vi "Quiz #3.vi"() -> ()   [LabVIEW 2017]
uses:
  Controlaleluya.ctl
  Maquinaestaleluya.ctl
  Control 2maqinestaaleluya.ctl
panel:
  out "array w/ subset deleted 4":string[][](array[string])
  out "spreadsheet string 4":string
  out "before substring 12":string
  out "match substring 12":string
  out "after substring 12":string
  out "text 8":string
  out "array 8":string[][](array[string])
  out "C.V 8":u8[](array[numeric])
  out "stop 16":bool
  out "C.V 7":u8[](array[numeric])
  out "stop 15":bool
  out "text 7":string
  out "array 7":string[][](array[string])
  out "element 8":string
  out "before substring 11":string
  out "match substring 11":string
  out "after substring 11":string
  out "element 7":string
  out "before substring 10":string
  out "match substring 10":string
  out "after substring 10":string
  in  "stop 14":bool
  in  "stop 13":bool
  out "Tab Control 2":enum32{"Loguin", "Usuarios", "Admin"}(tab)
  in  "Loguin 2":bool
  in  "Contraseña 4":string
  in  "Usuario 4":string
  in  "Nombre 4":string
  in  "Clave 4":string
  in  "Aceptar 4":bool
  out "OK Button 3":bool
  in  "Ingresar 2":bool
  in  "Borrar 2":bool
  in  "Clave/ingress 4":string
  in  "Usua/Ingress 4":string
  in  "Usuarios D/B 4":string[](array[string])
  out "mayu 2":i32
  out "min 2":i32
  in  "Salir 2":bool
  out "appended path 2":path
  in  "stop 3":bool
  in  "Salir":bool
  out "array 2":string[][](array[string])
  out "text 2":string
  out "appended path":path
  out "array w/ subset deleted":string[][](array[string])
  out "spreadsheet string":string
  out "after substring 3":string
  out "match substring 3":string
  out "before substring 3":string
  out "C.V":u8[](array[numeric])
  out "stop 4":bool
  out "C.V 2":u8[](array[numeric])
  out "mayu":i32
  out "min":i32
  out "stop 2":bool
  out "after substring 2":string
  out "match substring 2":string
  out "before substring 2":string
  out "element 2":string
  out "after substring":string
  out "match substring":string
  out "before substring":string
  out "element":string
  out "array":string[][](array[string])
  out "text":string
  in  "stop":bool
  out "Tab Control":enum32{"Loguin", "Usuarios", "Admin"}(tab)
  in  "Usuario":string
  in  "Contraseña":string
  in  "Loguin":bool
  out "OK Button":bool
  in  "Clave":string
  in  "Nombre":string
  in  "Aceptar":bool
  out "OK Button 2":bool
  in  "Ingresar":bool
  in  "Usua/Ingress":string
  in  "Clave/ingress":string
  in  "Borrar":bool
  in  "Usuarios D/B":string[](array[string])
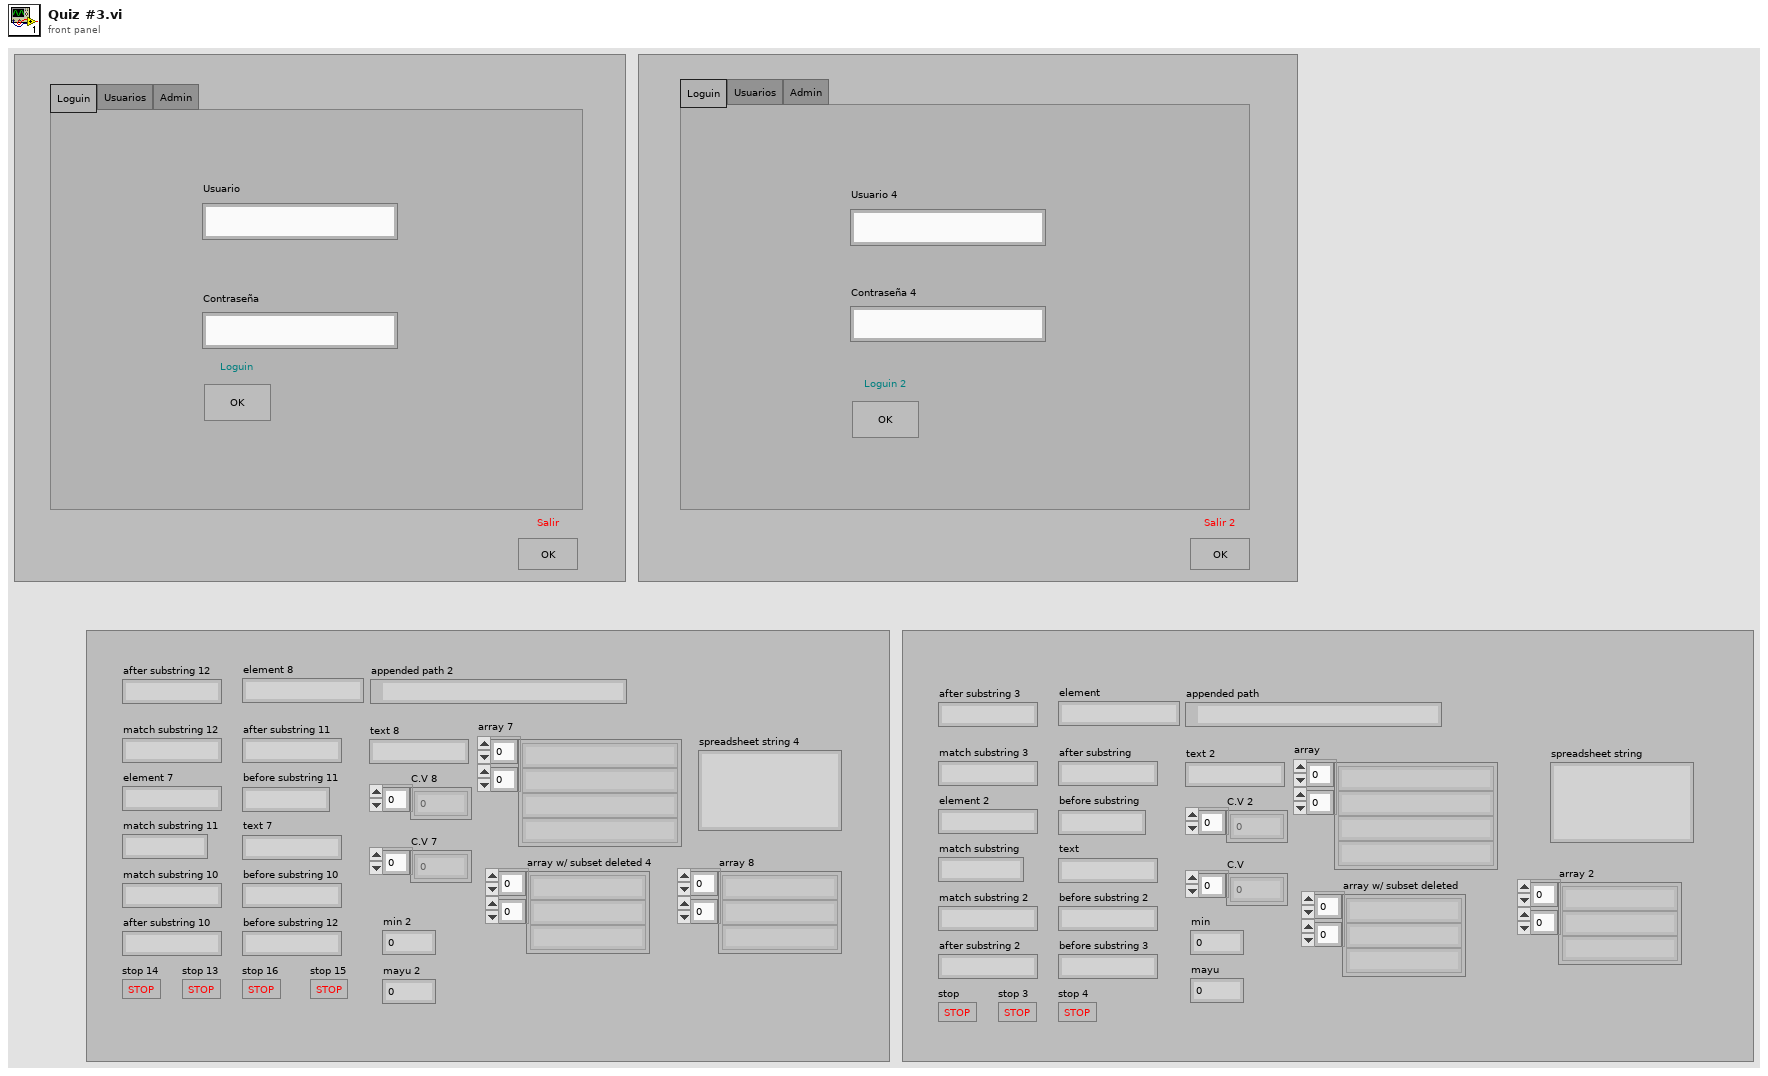
[diagram p1: front panel]
types:
  T1 = enum16{"open", "replace", "create", "open or create", "replace or create", "replace or create with confirmation"}
  T2 = typedef "Controlaleluya.ctl" = enum16{"Loguin", "Usuarios", "Admin"}
  T3 = typedef "Maquinaestaleluya.ctl" = enum16{"Control", "V.Usuario/Contraseña", "V.entre 8 y 16", "V.min y MAY", "ingresar"}
  T4 = typedef "Control 2maqinestaaleluya.ctl" = enum16{"Control", "V.Usuario/Contraseña", "V.Entre 8 y 16", "V.min y MAY", "Aceptar"}
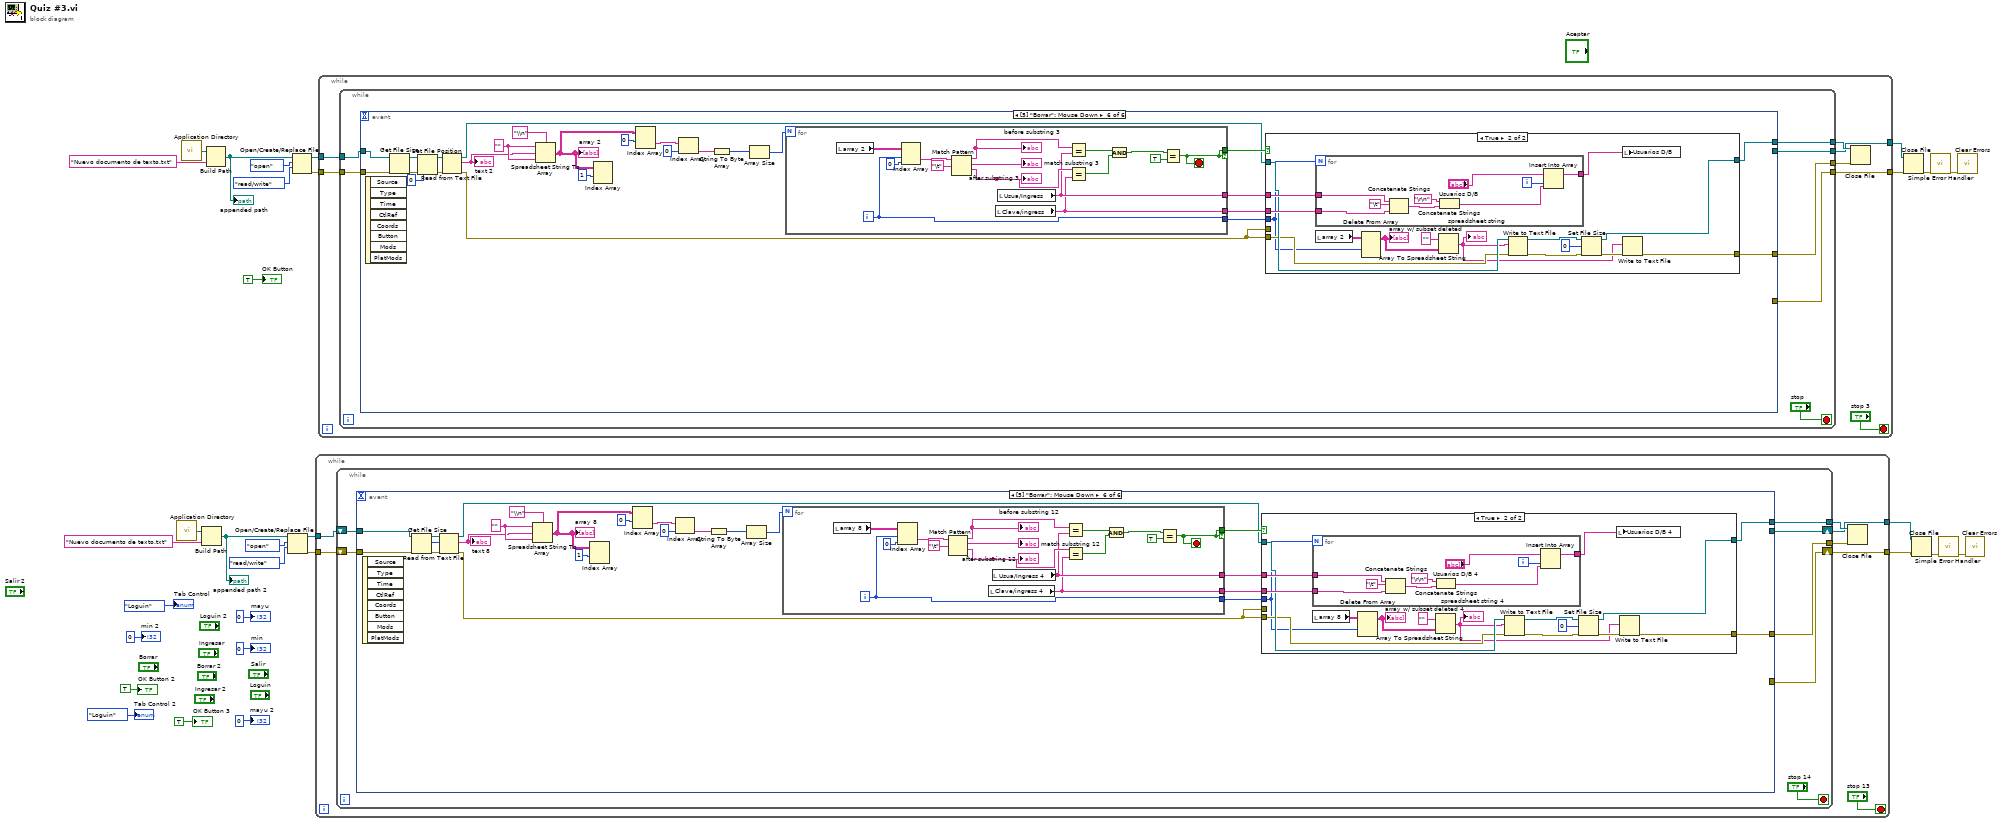
[diagram p0: block diagram]
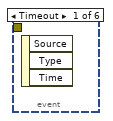
[diagram p2: hidden frame]
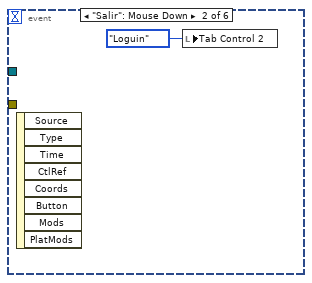
[diagram p3: hidden frame]
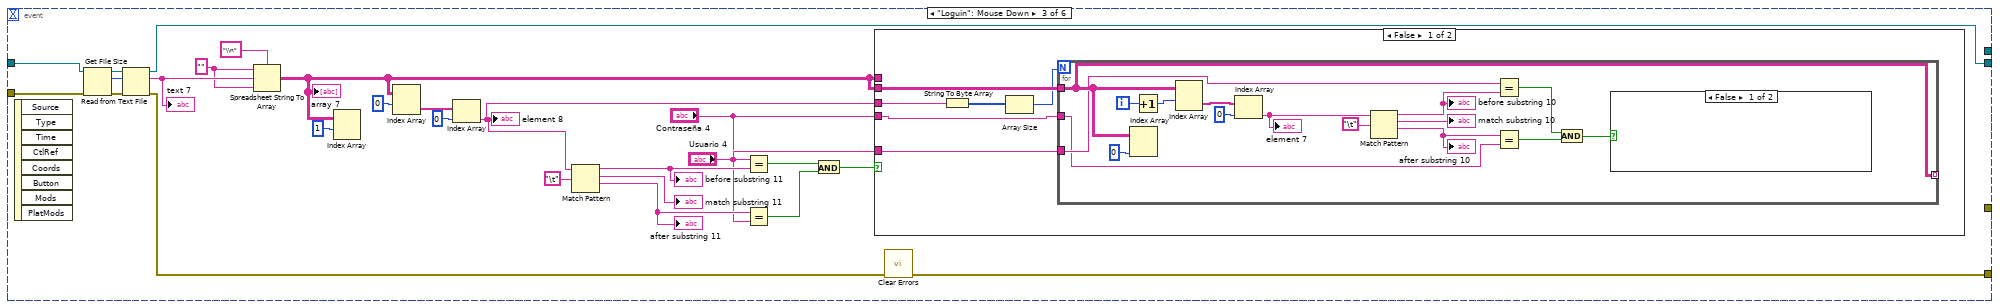
[diagram p4: hidden frame]
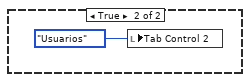
[diagram p5: hidden frame]
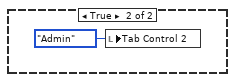
[diagram p6: hidden frame]
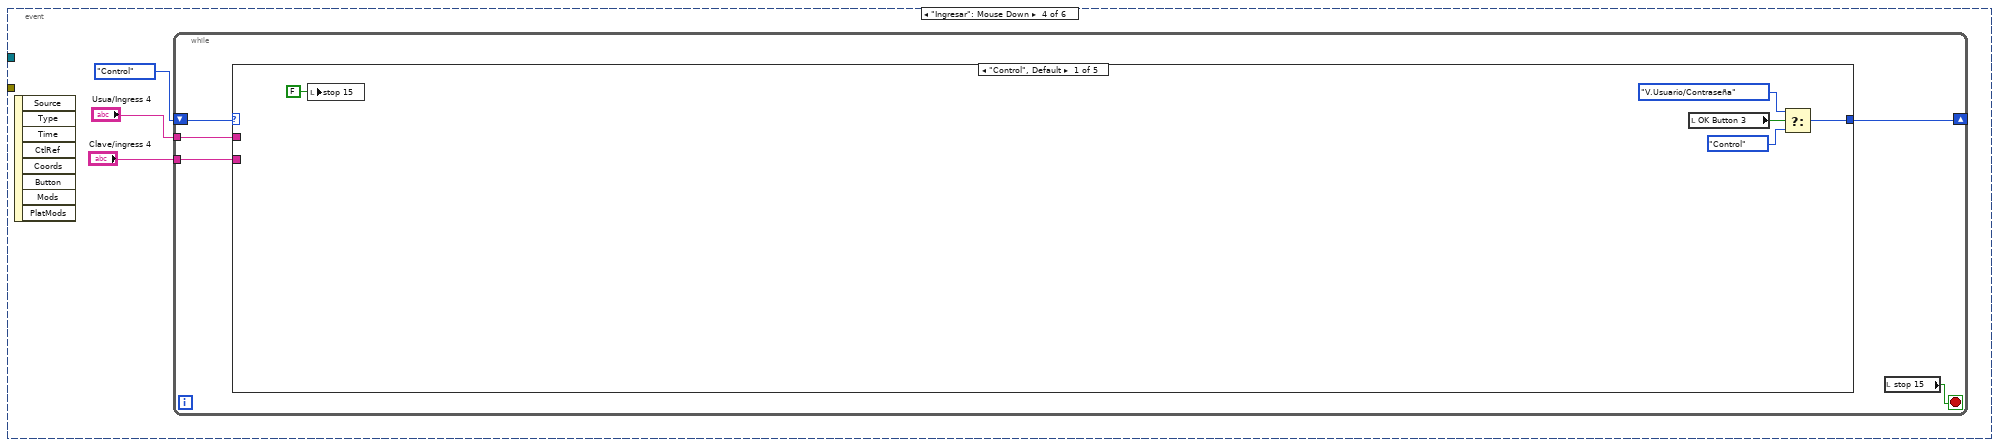
[diagram p7: hidden frame]
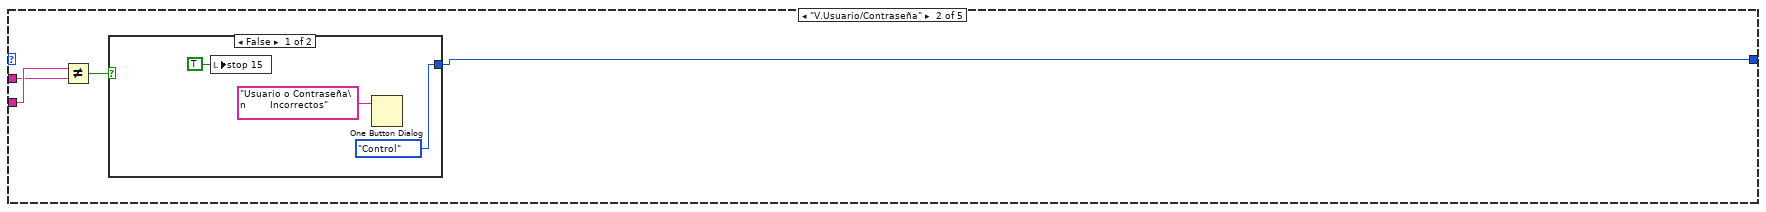
[diagram p8: hidden frame]
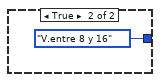
[diagram p9: hidden frame]
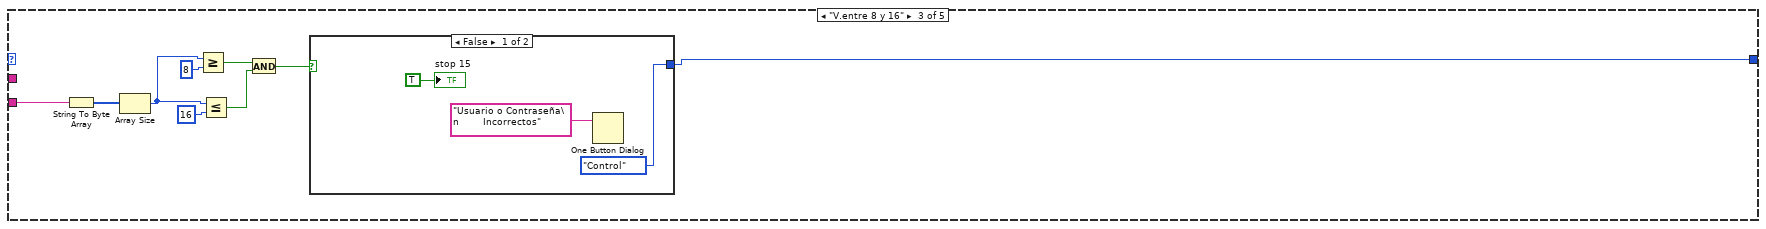
[diagram p10: hidden frame]
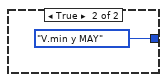
[diagram p11: hidden frame]
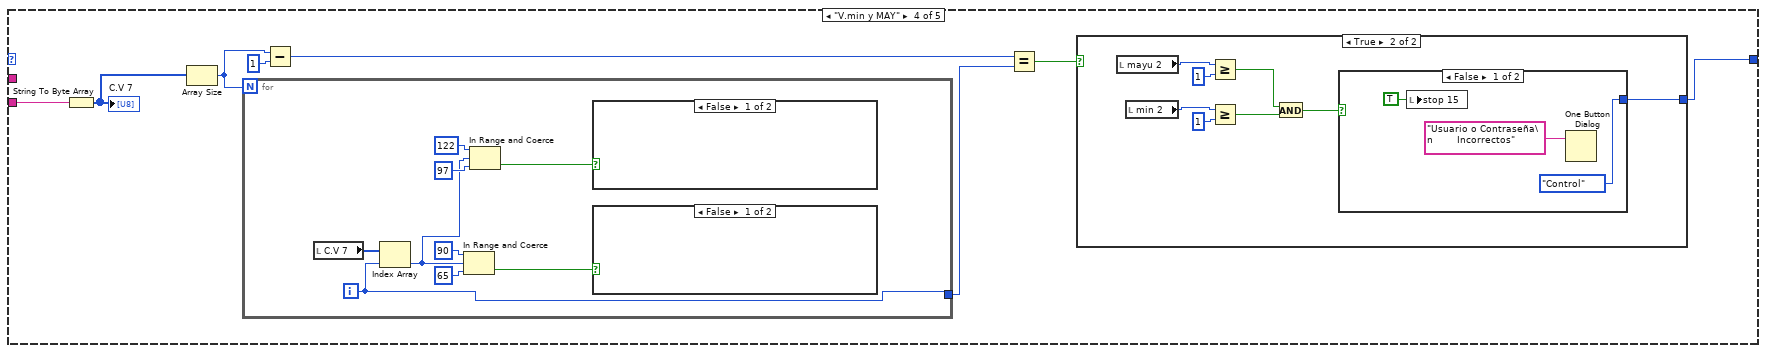
[diagram p12: hidden frame]
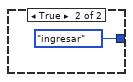
[diagram p14: hidden frame]
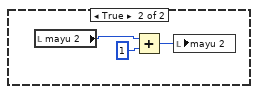
[diagram p15: hidden frame]
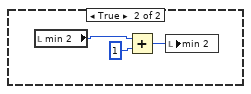
[diagram p16: hidden frame]
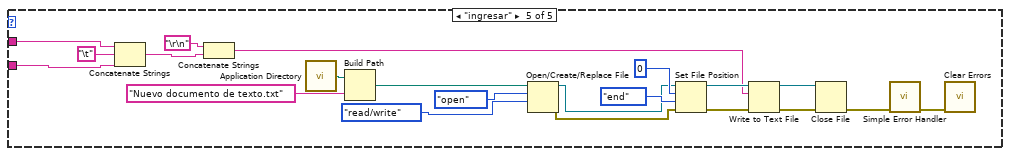
[diagram p17: hidden frame]
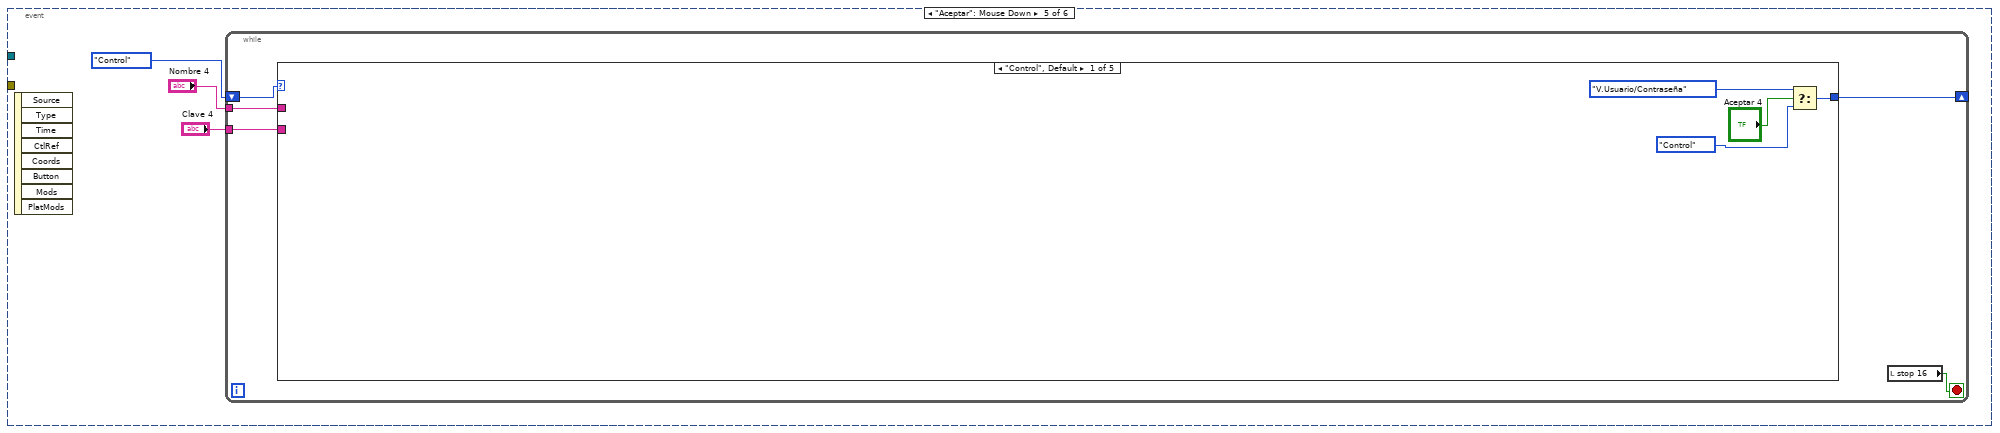
[diagram p18: hidden frame]
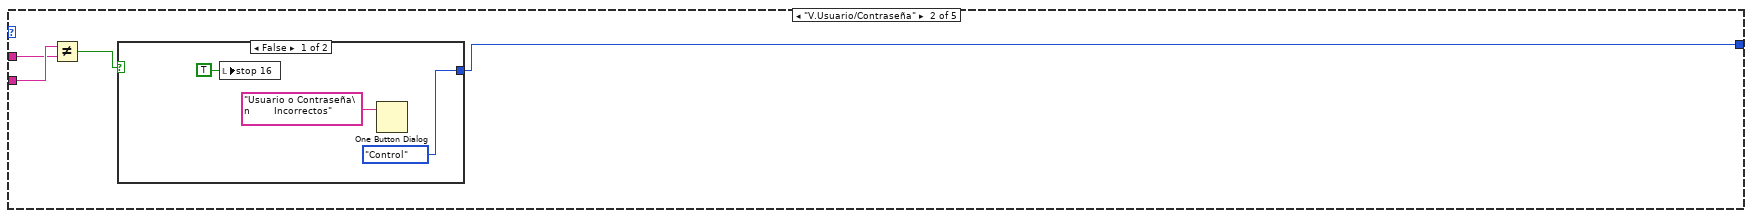
[diagram p19: hidden frame]
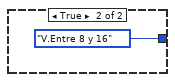
[diagram p20: hidden frame]
diagram:
  n1 = call <vilib>:"Application Directory.vi"() -> ("Application Directory"=w11:path)
  n2 = call <vilib>:"Application Directory.vi"() -> ("Application Directory"=w24:path)
  n3 = Build Path(base path=w11, name or relative path="Nuevo documento de texto.txt") -> (appended path=w13:path)
  "appended path 2" <- w13
  n4 = Build Path(base path=w24, name or relative path="Nuevo documento de texto.txt") -> (appended path=w22:path)
  "appended path" <- w22
  n5 = Open/Create/Replace File(file path (use dialog)=w13, operation (0:open)=T1."open", access (0:read/write)=enum16{"read/write", "read-only", "write-only"}."read/write") -> (refnum out=w5:refnum<file>, error out=w4:errorcluster)  [unwired: 3 in, 1 out]
  n6 = Open/Create/Replace File(file path (use dialog)=w22, operation (0:open)=T1."open", access (0:read/write)=enum16{"read/write", "read-only", "write-only"}."read/write") -> (refnum out=w26:refnum<file>, error out=w25:errorcluster)  [unwired: 3 in, 1 out]
  n7 = while {
    tunnel: w5 -> [w38]
    tunnel: w4 -> [w37]
    tunnel: [w34] -> w2
    tunnel: [w33] -> w3
    stop <- "stop 13" stop-if-true
    n8 = while {
      tunnel: [w44] -> w36
      tunnel: [w43] -> w35
      shift-right: [w40] -> w33
      shift-left: w38 -> [w42]
      shift-right: [w41] -> w34
      shift-left: w37 -> [w39]
      stop <- "stop 14" stop-if-true
      n9 = event shown="[5] \"Borrar\": Mouse Down" {
        selector: _ -> [_ _ _ _ _ _]
        dyn-events: _ -> [_ _ _ _ _ _]
        timeout: _ -> [_ _ _ _ _ _]
        tunnel: [_ _ w69 _ _ _] -> w41
        tunnel: [_ _ w57 _ _ _] -> w40
        tunnel: w42 -> [_ _ w51 _ _ w293]
        tunnel: w39 -> [_ _ w53 _ _ w292]
        tunnel: [_ _ _ _ _ w286] -> w44
        tunnel: [_ _ _ _ _ w285] -> w43
        event Timeout {
          n10 = event-data() -> ()  [unwired: 1 in, 3 out]
        }
        event "Salir": Mouse Down {
          n11 = event-data() -> ()  [unwired: 1 in, 8 out]
          n12 = local write "Tab Control 2"(Controlaleluya."Loguin") -> ()
        }
        event "Loguin": Mouse Down {
          w59 = "" ("array type (2D Dbl)")
          n13 = event-data() -> ()  [unwired: 1 in, 8 out]
          n14 = Get File Size(file=w51, error in=w53) -> (refnum out=w52:refnum<file>, size (in bytes)=w71:i64, 0:w72:errorcluster)
          n15 = Read from Text File(file (use dialog)=w52, count=w71, error in=w72) -> (refnum out=w57:refnum<file>, text=w68:string, error out=w70:errorcluster)  [unwired: 1 in, 1 out]
          "text 7" <- w68
          n16 = Spreadsheet String To Array(delimiter (Tab)="\\n", format string=w59, spreadsheet string=w68, array type (2D Dbl)=w59) -> (array=w50:string[][])
          "array 7" <- w50
          n17 = Index Array(array=w50, index (row)=1 ("index")) -> ()  [unwired: 1 in, 1 out]
          n18 = Index Array(array=w50, index (row)=0) -> (element=w64:string[])  [unwired: 1 in]
          n19 = Index Array(array=w64, index=0) -> (element=w56:string)
          "element 8" <- w56
          n20 = Match Pattern(string=w56, regular expression="\t") -> (before substring=w58:string, match substring=→"match substring 11":string, after substring=w60:string)  [unwired: 1 in, 1 out]
          "before substring 11" <- w58
          "after substring 11" <- w60
          n21 = Equal?(x="Usuario 4", y=w58) -> (x = y?=w49:bool)
          n22 = Equal?(x=w60, y="Contraseña 4") -> (x = y?=w48:bool)
          n23 = And(x=w49, y=w48) -> (x .and. y?=w47:bool)
          n24 = case shown="False" w47 {
            tunnel: w50 -> [_ _]
            tunnel: w50 -> [w78 _]
            tunnel: w56 -> [w77 _]
            tunnel: "Usuario 4" -> [w75 _]
            tunnel: "Contraseña 4" -> [w74 _]
            frame False {
              n25 = String To Byte Array(string=w77) -> (unsigned byte array=w76:u8[])
              n26 = Array Size(array=w76) -> (size(s)=w73:i32)
              n27 = for {
                N: w73 -> [_]
                tunnel: w78 -> [w83]
                tunnel: [w83] -> _ mode=indexing
                tunnel: w75 -> [w82]
                tunnel: w74 -> [w81]
                i -> [w80]
                n28 = Index Array(array=w83, index (col)=0) -> ()  [unwired: 1 in, 1 out]
                n29 = Increment(x=w80) -> (x+1=w79:i32)
                n30 = Index Array(array=w83, index (row)=w79) -> (element=w92:string[])  [unwired: 1 in]
                n31 = Index Array(array=w92, index=0) -> (element=w91:string)
                "element 7" <- w91
                n32 = Match Pattern(string=w91, regular expression="\t") -> (before substring=w89:string, match substring=→"match substring 10":string, after substring=w87:string)  [unwired: 1 in, 1 out]
                "before substring 10" <- w89
                "after substring 10" <- w87
                n33 = Equal?(x=w82, y=w89) -> (x = y?=w85:bool)
                n34 = Equal?(x=w87, y=w81) -> (x = y?=w86:bool)
                n35 = And(x=w85, y=w86) -> (x .and. y?=w84:bool)
                n36 = case shown="False" w84 {
                  frame False {
                  }
                  frame True {
                    n37 = local write "Tab Control 2"(Controlaleluya."Usuarios") -> ()
                  }
                }
              }
            }
            frame True {
              n38 = local write "Tab Control 2"(Controlaleluya."Admin") -> ()
            }
          }
          n39 = call <vilib>:"Clear Errors.vi"("error in (no error)"=w70) -> ("error out"=w69:errorcluster)  [unwired: 5 in, 1 out]
        }
        event "Ingresar": Mouse Down {
          n40 = event-data() -> ()  [unwired: 1 in, 8 out]
          n41 = while {
            tunnel: "Usua/Ingress 4" -> [w104]
            shift-right: [w102] -> _
            shift-left: Maquinaestaleluya."Control" -> [w103]
            tunnel: "Clave/ingress 4" -> [w101]
            stop <- w100 stop-if-true
            n42 = case shown="\"Control\", Default" w103 {
              tunnel: w104 -> [_ w112 _ _ w167]
              tunnel: w101 -> [_ w113 w126 w138 w168]
              tunnel: [w109 w110 w124 w132 _] -> w102
              frame "Control", Default {
                n43 = local write "stop 15"(FALSE) -> ()
                n44 = local read "OK Button 3"() -> (w106:bool)
                n45 = Select(t=Maquinaestaleluya."V.Usuario/Contraseña", s=w106, f=Maquinaestaleluya."Control") -> (s? t:f=w109:T3)
              }
              frame "V.Usuario/Contraseña" {
                n46 = Not Equal?(x=w113, y=w112) -> (x != y?=w111:bool)
                n47 = case shown="False" w111 {
                  tunnel: [Maquinaestaleluya."Control" Maquinaestaleluya."V.entre 8 y 16"] -> w110
                  frame False {
                    n48 = local write "stop 15"(TRUE) -> ()
                    n49 = One Button Dialog(message="Usuario o Contraseña\n        Incorrectos") -> ()  [unwired: 1 in, 1 out]
                  }
                  frame True {
                  }
                }
              }
              frame "V.entre 8 y 16" {
                n50 = String To Byte Array(string=w126) -> (unsigned byte array=w125:u8[])
                n51 = Array Size(array=w125) -> (size(s)=w121:i32)
                n52 = Greater Or Equal?(x=w121, y=8) -> (x >= y?=w120:bool)
                n53 = Less Or Equal?(x=w121, y=16) -> (x <= y?=w119:bool)
                n54 = And(x=w120, y=w119) -> (x .and. y?=w118:bool)
                n55 = case shown="False" w118 {
                  tunnel: [Maquinaestaleluya."Control" Maquinaestaleluya."V.min y MAY"] -> w124
                  frame False {
                    n56 = One Button Dialog(message="Usuario o Contraseña\n        Incorrectos") -> ()  [unwired: 1 in, 1 out]
                    "stop 15" <- TRUE
                  }
                  frame True {
                  }
                }
              }
              frame "V.min y MAY" {
                n57 = String To Byte Array(string=w138) -> (unsigned byte array=w131:u8[])
                "C.V 7" <- w131
                n58 = Array Size(array=w131) -> (size(s)=w135:i32)
                n59 = for {
                  N: w135 -> [_]
                  tunnel: [w153] -> w137
                  i -> [w153]
                  n60 = local read "C.V 7"() -> (w151:u8[])
                  n61 = Index Array(array=w151, index=w153) -> (element=w155:u8)
                  n62 = In Range and Coerce(upper limit=90, x=w155, lower limit=65) -> (In Range?=w152:bool)  [unwired: 1 out]
                  n63 = In Range and Coerce(upper limit=122, x=w155, lower limit=97) -> (In Range?=w154:bool)  [unwired: 1 out]
                  n64 = case shown="False" w154 {
                    frame False {
                    }
                    frame True {
                      n65 = local read "min 2"() -> (w165:i32)
                      n66 = Add(x=w165, y=1) -> (x+y=w164:i32)
                      n67 = local write "min 2"(w164) -> ()
                    }
                  }
                  n68 = case shown="False" w152 {
                    frame False {
                    }
                    frame True {
                      n69 = local read "mayu 2"() -> (w162:i32)
                      n70 = Add(x=w162, y=1) -> (x+y=w161:i32)
                      n71 = local write "mayu 2"(w161) -> ()
                    }
                  }
                }
                n72 = Subtract(x=w135, y=1) -> (x-y=w136:i32)
                n73 = Equal?(x=w136, y=w137) -> (x = y?=w133:bool)
                n74 = case shown="True" w133 {
                  tunnel: [_ w145] -> w132
                  frame False {
                  }
                  frame True {
                    n75 = local read "mayu 2"() -> (w142:i32)
                    n76 = local read "min 2"() -> (w140:i32)
                    n77 = Greater Or Equal?(x=w142, y=1 ("x")) -> (x >= y?=w144:bool)
                    n78 = Greater Or Equal?(x=w140, y=1 ("x")) -> (x >= y?=w143:bool)
                    n79 = And(x=w144, y=w143) -> (x .and. y?=w146:bool)
                    n80 = case shown="False" w146 {
                      tunnel: [Maquinaestaleluya."Control" Maquinaestaleluya."ingresar"] -> w145
                      frame False {
                        n81 = local write "stop 15"(TRUE) -> ()
                        n82 = One Button Dialog(message="Usuario o Contraseña\n        Incorrectos") -> ()  [unwired: 1 in, 1 out]
                      }
                      frame True {
                      }
                    }
                  }
                }
              }
              frame "ingresar" {
                n83 = Concatenate Strings(w167, "\t", w168) -> (w178:string)
                n84 = Concatenate Strings("\r\n", w178) -> (w169:string)
                n85 = call <vilib>:"Application Directory.vi"() -> ("Application Directory"=w170:path)
                n86 = Build Path(base path=w170, name or relative path="Nuevo documento de texto.txt") -> (appended path=w171:path)
                n87 = Open/Create/Replace File(file path (use dialog)=w171, operation (0:open)=T1."open", access (0:read/write)=enum16{"read/write", "read-only", "write-only"}."read/write") -> (refnum out=w172:refnum<file>, error out=w173:errorcluster)  [unwired: 3 in, 1 out]
                n88 = Set File Position(offset (in bytes) (0)=i64 0, refnum=w172, from (0:start)=enum16{"start", "end", "current"}."end", error in=w173) -> (refnum out=w180:refnum<file>, error out=w174:errorcluster)
                n89 = Write to Text File(file (use dialog)=w180, text=w169, error in=w174) -> (refnum out=w177:refnum<file>, error out=w179:errorcluster)  [unwired: 1 in, 1 out]
                n90 = Close File(refnum=w177, error in=w179) -> (error out=w176:errorcluster)  [unwired: 1 out]
                n91 = call <vilib>:"Simple Error Handler.vi"("error in (no error)"=w176) -> ("error out"=w175:errorcluster)  [unwired: 4 in, 4 out]
                n92 = call <vilib>:"Clear Errors.vi"("error in (no error)"=w175) -> ()  [unwired: 5 in, 2 out]
              }
            }
            n93 = local read "stop 15"() -> (w100:bool)
          }
        }
        event "Aceptar": Mouse Down {
          n94 = event-data() -> ()  [unwired: 1 in, 8 out]
          n95 = while {
            tunnel: "Clave 4" -> [w194]
            tunnel: "Nombre 4" -> [w193]
            shift-right: [w191] -> _
            shift-left: Control_2maqinestaaleluya."Control" -> [w192]
            stop <- w190 stop-if-true
            n96 = case shown="\"Control\", Default" w192 {
              tunnel: w194 -> [_ w202 w209 w221 w257]
              tunnel: w193 -> [_ w201 _ _ w256]
              tunnel: [w195 w199 w207 w220 _] -> w191
              frame "Control", Default {
                n97 = Select(t=Control_2maqinestaaleluya."V.Usuario/Contraseña", s="Aceptar 4", f=Control_2maqinestaaleluya."Control") -> (s? t:f=w195:T4)
              }
              frame "V.Usuario/Contraseña" {
                n98 = Not Equal?(x=w202, y=w201) -> (x != y?=w200:bool)
                n99 = case shown="False" w200 {
                  tunnel: [Control_2maqinestaaleluya."Control" Control_2maqinestaaleluya."V.Entre 8 y 16"] -> w199
                  frame False {
                    n100 = local write "stop 16"(TRUE) -> ()
                    n101 = One Button Dialog(message="Usuario o Contraseña\n        Incorrectos") -> ()  [unwired: 1 in, 1 out]
                  }
                  frame True {
                  }
                }
              }
              frame "V.Entre 8 y 16" {
                n102 = String To Byte Array(string=w209) -> (unsigned byte array=w210:u8[])
                n103 = Array Size(array=w210) -> (size(s)=w211:i32)
                n104 = Greater Or Equal?(x=w211, y=8) -> (x >= y?=w214:bool)
                n105 = Less Or Equal?(x=w211, y=16) -> (x <= y?=w215:bool)
                n106 = And(x=w214, y=w215) -> (x .and. y?=w208:bool)
                n107 = case shown="False" w208 {
                  tunnel: [Control_2maqinestaaleluya."Control" Control_2maqinestaaleluya."V.min y MAY"] -> w207
                  frame False {
                    n108 = One Button Dialog(message="Usuario o Contraseña\n        Incorrectos") -> ()  [unwired: 1 in, 1 out]
                    "stop 16" <- TRUE
                  }
                  frame True {
                  }
                }
              }
              frame "V.min y MAY" {
                n109 = String To Byte Array(string=w221) -> (unsigned byte array=w226:u8[])
                "C.V 8" <- w226
                n110 = Array Size(array=w226) -> (size(s)=w223:i32)
                n111 = for {
                  N: w223 -> [_]
                  tunnel: [w241] -> w225
                  i -> [w241]
                  n112 = local read "C.V 8"() -> (w244:u8[])
                  n113 = Index Array(array=w244, index=w241) -> (element=w243:u8)
                  n114 = In Range and Coerce(upper limit=90, x=w243, lower limit=65) -> (In Range?=w240:bool)  [unwired: 1 out]
                  n115 = In Range and Coerce(upper limit=122, x=w243, lower limit=97) -> (In Range?=w242:bool)  [unwired: 1 out]
                  n116 = case shown="False" w242 {
                    frame False {
                    }
                    frame True {
                      n117 = local read "min 2"() -> (w254:i32)
                      n118 = Add(x=w254, y=1) -> (x+y=w253:i32)
                      n119 = local write "min 2"(w253) -> ()
                    }
                  }
                  n120 = case shown="False" w240 {
                    frame False {
                    }
                    frame True {
                      n121 = local read "mayu 2"() -> (w251:i32)
                      n122 = Add(x=w251, y=1) -> (x+y=w250:i32)
                      n123 = local write "mayu 2"(w250) -> ()
                    }
                  }
                }
                n124 = Subtract(x=w223, y=1) -> (x-y=w224:i32)
                n125 = Equal?(x=w224, y=w225) -> (x = y?=w222:bool)
                n126 = case shown="True" w222 {
                  tunnel: [_ w234] -> w220
                  frame False {
                  }
                  frame True {
                    n127 = local read "mayu 2"() -> (w228:i32)
                    n128 = local read "min 2"() -> (w231:i32)
                    n129 = Greater Or Equal?(x=w228, y=1 ("x")) -> (x >= y?=w233:bool)
                    n130 = Greater Or Equal?(x=w231, y=1 ("x")) -> (x >= y?=w232:bool)
                    n131 = And(x=w233, y=w232) -> (x .and. y?=w235:bool)
                    n132 = case shown="False" w235 {
                      tunnel: [Control_2maqinestaaleluya."Control" Control_2maqinestaaleluya."Aceptar"] -> w234
                      frame False {
                        n133 = local write "stop 16"(TRUE) -> ()
                        n134 = One Button Dialog(message="Usuario o Contraseña\n        Incorrectos") -> ()  [unwired: 1 in, 1 out]
                      }
                      frame True {
                      }
                    }
                  }
                }
              }
              frame "Aceptar" {
                n135 = Concatenate Strings(w256, "\t", w257) -> (w270:string)
                n136 = Concatenate Strings("\n", w270) -> (w275:string)
                n137 = call <vilib>:"Application Directory.vi"() -> ("Application Directory"=w268:path)
                n138 = Build Path(base path=w268, name or relative path="Nuevo documento de texto.txt") -> (appended path=w269:path)
                n139 = Open/Create/Replace File(file path (use dialog)=w269, operation (0:open)=T1."open", access (0:read/write)=enum16{"read/write", "read-only", "write-only"}."read/write") -> (refnum out=w266:refnum<file>, error out=w267:errorcluster)  [unwired: 3 in, 1 out]
                n140 = Set File Position(offset (in bytes) (0)=i64 0, refnum=w266, from (0:start)=enum16{"start", "end", "current"}."end", error in=w267) -> (refnum out=w274:refnum<file>, error out=w271:errorcluster)
                n141 = Write to Text File(file (use dialog)=w274, text=w275, error in=w271) -> (refnum out=w273:refnum<file>, error out=w272:errorcluster)  [unwired: 1 in, 1 out]
                n142 = Close File(refnum=w273, error in=w272) -> (error out=w265:errorcluster)  [unwired: 1 out]
                n143 = call <vilib>:"Simple Error Handler.vi"("error in (no error)"=w265) -> ("error out"=w264:errorcluster)  [unwired: 4 in, 4 out]
                n144 = call <vilib>:"Clear Errors.vi"("error in (no error)"=w264) -> ()  [unwired: 5 in, 2 out]
              }
            }
            n145 = local read "stop 16"() -> (w190:bool)
          }
        }
        event "Borrar": Mouse Down {
          w281 = "" ("format string")
          n146 = event-data() -> ()  [unwired: 1 in, 8 out]
          n147 = Get File Size(file=w293, error in=w292) -> (refnum out=w290:refnum<file>, size (in bytes)=w291:i64, 0:w289:errorcluster)
          n148 = Read from Text File(file (use dialog)=w290, count=w291, error in=w289) -> (refnum out=w288:refnum<file>, text=w280:string, error out=w287:errorcluster)  [unwired: 1 in, 1 out]
          "text 8" <- w280
          n149 = Spreadsheet String To Array(delimiter (Tab)="\\n", format string=w281, spreadsheet string=w280, array type (2D Dbl)=w281) -> (array=w279:string[][])
          "array 8" <- w279
          n150 = Index Array(array=w279, index (row)=1) -> ()  [unwired: 1 in, 1 out]
          n151 = Index Array(array=w279, index (row)=0) -> (element=w278:string[])  [unwired: 1 in]
          n152 = Index Array(array=w278, index=0) -> (element=w276:string)
          n153 = String To Byte Array(string=w276) -> (unsigned byte array=w298:u8[])
          n154 = Array Size(array=w298) -> (size(s)=w299:i32)
          n155 = for {
            N: w299 -> [_]
            tunnel: [w304] -> w297 if=w304
            tunnel: [w303] -> w296
            tunnel: [w302] -> w295
            tunnel: [w301] -> w294
            i -> [w301]
            stop <- w304 stop-if-true
            n156 = local read "array 8"() -> (w300:string[][])
            n157 = Index Array(array=w300, index (row)=w301, index (col)=0 ("disabled index (col)")) -> (element=w313:string)
            n158 = Match Pattern(string=w313, regular expression="\t") -> (before substring=w309:string, match substring=→"match substring 12":string, after substring=w310:string)  [unwired: 1 in, 1 out]
            "before substring 12" <- w309
            "after substring 12" <- w310
            n159 = local read "Clave/ingress 4"() -> (w302:string)
            n160 = local read "Usua/Ingress 4"() -> (w303:string)
            n161 = Equal?(x=w309, y=w303) -> (x = y?=w308:bool)
            n162 = Equal?(x=w310, y=w302) -> (x = y?=w307:bool)
            n163 = And(x=w308, y=w307) -> (x .and. y?=w306:bool)
            n164 = Equal?(x=w306, y=TRUE) -> (x = y?=w304:bool)
          }
          n165 = case shown="True" w297 {
            tunnel: w296 -> [_ w329]
            tunnel: w295 -> [_ w330]
            tunnel: w294 -> [_ w315]
            tunnel: w288 -> [_ w323]
            tunnel: [_ w319] -> w285
            tunnel: [_ w317] -> w286
            tunnel: w287 -> [_ w322]
            tunnel: w287 -> [_ _]
            frame False {
            }
            frame True {
              n166 = for {
                N: w315 -> [_]
                tunnel: w330 -> [w337]
                tunnel: w329 -> [w339]
                tunnel: [w333] -> w328
                i -> [w332]
                n167 = Concatenate Strings(w339, "\t", w337) -> (w335:string)
                n168 = Concatenate Strings("\r\n", w335) -> (w331:string)
                n169 = Insert Into Array(array="Usuarios D/B 4", index=w332, new element=w331) -> (w333:string[])
              }
              n170 = local read "array 8"() -> (w321:string[][])
              n171 = Delete From Array(array=w321, index (row)=w315) -> (array with subset deleted=w327:string[][])  [unwired: 2 in, 1 out]
              "array w/ subset deleted 4" <- w327
              n172 = Array To Spreadsheet String(array=w327, 3:"" ("format string")) -> (spreadsheet string=w316:string)  [unwired: 1 in]
              "spreadsheet string 4" <- w316
              n173 = Write to Text File(file (use dialog)=w323, text=w316, error in=w322) -> (refnum out=w320:refnum<file>, error out=w324:errorcluster)  [unwired: 1 in, 1 out]
              n174 = Set File Size(4:w324, 6:i64 0 ("size (in bytes)"), 7:w320) -> (0:w318:errorcluster, 3:w319:refnum<file>)
              n175 = local write "Usuarios D/B 4"(w328) -> ()
              n176 = Write to Text File(text=w316, error in=w318) -> (error out=w317:errorcluster)  [unwired: 2 in, 2 out]
            }
          }
        }
      }
    }
    n177 = Close File(refnum=w35, error in=w36) -> ()  [unwired: 2 out]
  }
  n178 = while {
    tunnel: w26 -> [w343]
    tunnel: w25 -> [w342]
    tunnel: [w341] -> w18
    tunnel: [w340] -> w17
    stop <- "stop 3" stop-if-true
    n179 = while {
      tunnel: [w352] -> w346
      tunnel: [w351] -> w345
      tunnel: w343 -> [w350]
      tunnel: w342 -> [w349]
      tunnel: [w348] -> w341
      tunnel: [w347] -> w340
      stop <- "stop" stop-if-true
      n180 = event shown="[5] \"Borrar\": Mouse Down" {
        selector: _ -> [_ _ _ _ _ _]
        dyn-events: _ -> [_ _ _ _ _ _]
        timeout: _ -> [_ _ _ _ _ _]
        tunnel: [_ _ w377 _ _ _] -> w348
        tunnel: [_ _ w365 _ _ _] -> w347
        tunnel: w350 -> [_ _ w359 _ _ w588]
        tunnel: w349 -> [_ _ w361 _ _ w606]
        tunnel: [_ _ _ _ _ w603] -> w352
        tunnel: [_ _ _ _ _ w602] -> w351
        event Timeout {
          n181 = event-data() -> ()  [unwired: 1 in, 3 out]
        }
        event "Salir": Mouse Down {
          n182 = event-data() -> ()  [unwired: 1 in, 8 out]
          n183 = local write "Tab Control"(Controlaleluya."Loguin") -> ()
        }
        event "Loguin": Mouse Down {
          w367 = "" ("array type (2D Dbl)")
          n184 = event-data() -> ()  [unwired: 1 in, 8 out]
          n185 = Get File Size(file=w359, error in=w361) -> (refnum out=w360:refnum<file>, size (in bytes)=w379:i64, 0:w380:errorcluster)
          n186 = Read from Text File(file (use dialog)=w360, count=w379, error in=w380) -> (refnum out=w365:refnum<file>, text=w376:string, error out=w378:errorcluster)  [unwired: 1 in, 1 out]
          "text" <- w376
          n187 = Spreadsheet String To Array(delimiter (Tab)="\\n", format string=w367, spreadsheet string=w376, array type (2D Dbl)=w367) -> (array=w358:string[][])
          "array" <- w358
          n188 = Index Array(array=w358, index (row)=1 ("index")) -> ()  [unwired: 1 in, 1 out]
          n189 = Index Array(array=w358, index (row)=0) -> (element=w372:string[])  [unwired: 1 in]
          n190 = Index Array(array=w372, index=0) -> (element=w364:string)
          "element" <- w364
          n191 = Match Pattern(string=w364, regular expression="\t") -> (before substring=w366:string, match substring=→"match substring":string, after substring=w368:string)  [unwired: 1 in, 1 out]
          "before substring" <- w366
          "after substring" <- w368
          n192 = Equal?(x="Usuario", y=w366) -> (x = y?=w357:bool)
          n193 = Equal?(x=w368, y="Contraseña") -> (x = y?=w356:bool)
          n194 = And(x=w357, y=w356) -> (x .and. y?=w355:bool)
          n195 = case shown="False" w355 {
            tunnel: w358 -> [_ _]
            tunnel: w358 -> [w386 _]
            tunnel: w364 -> [w385 _]
            tunnel: "Usuario" -> [w383 _]
            tunnel: "Contraseña" -> [w382 _]
            frame False {
              n196 = String To Byte Array(string=w385) -> (unsigned byte array=w384:u8[])
              n197 = Array Size(array=w384) -> (size(s)=w381:i32)
              n198 = for {
                N: w381 -> [_]
                tunnel: w386 -> [w391]
                tunnel: [w391] -> _ mode=indexing
                tunnel: w383 -> [w390]
                tunnel: w382 -> [w389]
                i -> [w388]
                n199 = Index Array(array=w391, index (col)=0) -> ()  [unwired: 1 in, 1 out]
                n200 = Increment(x=w388) -> (x+1=w387:i32)
                n201 = Index Array(array=w391, index (row)=w387) -> (element=w400:string[])  [unwired: 1 in]
                n202 = Index Array(array=w400, index=0) -> (element=w399:string)
                "element 2" <- w399
                n203 = Match Pattern(string=w399, regular expression="\t") -> (before substring=w397:string, match substring=→"match substring 2":string, after substring=w395:string)  [unwired: 1 in, 1 out]
                "before substring 2" <- w397
                "after substring 2" <- w395
                n204 = Equal?(x=w390, y=w397) -> (x = y?=w393:bool)
                n205 = Equal?(x=w395, y=w389) -> (x = y?=w394:bool)
                n206 = And(x=w393, y=w394) -> (x .and. y?=w392:bool)
                n207 = case shown="True" w392 {
                  frame False {
                  }
                  frame True {
                    n208 = local write "Tab Control"(Controlaleluya."Usuarios") -> ()
                  }
                }
              }
            }
            frame True {
              n209 = local write "Tab Control"(Controlaleluya."Admin") -> ()
            }
          }
          n210 = call <vilib>:"Clear Errors.vi"("error in (no error)"=w378) -> ("error out"=w377:errorcluster)  [unwired: 5 in, 1 out]
        }
        event "Ingresar": Mouse Down {
          n211 = event-data() -> ()  [unwired: 1 in, 8 out]
          n212 = while {
            tunnel: "Usua/Ingress" -> [w412]
            tunnel: "Clave/ingress" -> [w411]
            shift-right: [w408] -> _
            shift-left: Maquinaestaleluya."Control" -> [w409]
            stop <- w410 stop-if-true
            n213 = case shown="\"ingresar\"" w409 {
              tunnel: w412 -> [_ w420 _ _ w476]
              tunnel: w411 -> [_ w421 w434 w446 w477]
              tunnel: [w413 w418 w426 w439 _] -> w408
              frame "Control", Default {
                n214 = local write "stop 2"(FALSE) -> ()
                n215 = local read "OK Button 2"() -> (w415:bool)
                n216 = Select(t=Maquinaestaleluya."V.Usuario/Contraseña", s=w415, f=Maquinaestaleluya."Control") -> (s? t:f=w413:T3)
              }
              frame "V.Usuario/Contraseña" {
                n217 = Not Equal?(x=w421, y=w420) -> (x != y?=w419:bool)
                n218 = case shown="True" w419 {
                  tunnel: [Maquinaestaleluya."Control" Maquinaestaleluya."V.entre 8 y 16"] -> w418
                  frame False {
                    n219 = local write "stop 2"(TRUE) -> ()
                    n220 = One Button Dialog(message="Usuario o Contraseña\n        Incorrectos") -> ()  [unwired: 1 in, 1 out]
                  }
                  frame True {
                  }
                }
              }
              frame "V.entre 8 y 16" {
                n221 = String To Byte Array(string=w434) -> (unsigned byte array=w433:u8[])
                n222 = Array Size(array=w433) -> (size(s)=w430:i32)
                n223 = Greater Or Equal?(x=w430, y=8) -> (x >= y?=w429:bool)
                n224 = Less Or Equal?(x=w430, y=16) -> (x <= y?=w428:bool)
                n225 = And(x=w429, y=w428) -> (x .and. y?=w427:bool)
                n226 = case shown="True" w427 {
                  tunnel: [Maquinaestaleluya."Control" Maquinaestaleluya."V.min y MAY"] -> w426
                  frame False {
                    n227 = One Button Dialog(message="Usuario o Contraseña\n        Incorrectos") -> ()  [unwired: 1 in, 1 out]
                    "stop 2" <- TRUE
                  }
                  frame True {
                  }
                }
              }
              frame "V.min y MAY" {
                n228 = String To Byte Array(string=w446) -> (unsigned byte array=w440:u8[])
                "C.V" <- w440
                n229 = Array Size(array=w440) -> (size(s)=w443:i32)
                n230 = for {
                  N: w443 -> [_]
                  tunnel: [w461] -> w445
                  i -> [w461]
                  n231 = local read "C.V"() -> (w459:u8[])
                  n232 = Index Array(array=w459, index=w461) -> (element=w463:u8)
                  n233 = In Range and Coerce(upper limit=90, x=w463, lower limit=65) -> (In Range?=w460:bool)  [unwired: 1 out]
                  n234 = In Range and Coerce(upper limit=122, x=w463, lower limit=97) -> (In Range?=w462:bool)  [unwired: 1 out]
                  n235 = case shown="False" w462 {
                    frame False {
                    }
                    frame True {
                      n236 = local read "min"() -> (w473:i32)
                      n237 = Add(x=w473, y=1) -> (x+y=w472:i32)
                      n238 = local write "min"(w472) -> ()
                    }
                  }
                  n239 = case shown="False" w460 {
                    frame False {
                    }
                    frame True {
                      n240 = local read "mayu"() -> (w470:i32)
                      n241 = Add(x=w470, y=1) -> (x+y=w469:i32)
                      n242 = local write "mayu"(w469) -> ()
                    }
                  }
                }
                n243 = Subtract(x=w443, y=1) -> (x-y=w444:i32)
                n244 = Equal?(x=w444, y=w445) -> (x = y?=w441:bool)
                n245 = case shown="True" w441 {
                  tunnel: [_ w453] -> w439
                  frame False {
                  }
                  frame True {
                    n246 = local read "mayu"() -> (w450:i32)
                    n247 = local read "min"() -> (w448:i32)
                    n248 = Greater Or Equal?(x=w450, y=1 ("x")) -> (x >= y?=w452:bool)
                    n249 = Greater Or Equal?(x=w448, y=1 ("x")) -> (x >= y?=w451:bool)
                    n250 = And(x=w452, y=w451) -> (x .and. y?=w454:bool)
                    n251 = case shown="False" w454 {
                      tunnel: [Maquinaestaleluya."Control" Maquinaestaleluya."ingresar"] -> w453
                      frame False {
                        n252 = local write "stop 2"(TRUE) -> ()
                        n253 = One Button Dialog(message="Usuario o Contraseña\n        Incorrectos") -> ()  [unwired: 1 in, 1 out]
                      }
                      frame True {
                      }
                    }
                  }
                }
              }
              frame "ingresar" {
                n254 = Concatenate Strings(w476, "\t", w477) -> (w487:string)
                n255 = Concatenate Strings("\r\n", w487) -> (w478:string)
                n256 = call <vilib>:"Application Directory.vi"() -> ("Application Directory"=w479:path)
                n257 = Build Path(base path=w479, name or relative path="Nuevo documento de texto.txt") -> (appended path=w480:path)
                n258 = Open/Create/Replace File(file path (use dialog)=w480, operation (0:open)=T1."open", access (0:read/write)=enum16{"read/write", "read-only", "write-only"}."read/write") -> (refnum out=w481:refnum<file>, error out=w482:errorcluster)  [unwired: 3 in, 1 out]
                n259 = Set File Position(offset (in bytes) (0)=i64 0, refnum=w481, from (0:start)=enum16{"start", "end", "current"}."end", error in=w482) -> (refnum out=w489:refnum<file>, error out=w483:errorcluster)
                n260 = Write to Text File(file (use dialog)=w489, text=w478, error in=w483) -> (refnum out=w486:refnum<file>, error out=w488:errorcluster)  [unwired: 1 in, 1 out]
                n261 = Close File(refnum=w486, error in=w488) -> (error out=w485:errorcluster)  [unwired: 1 out]
                n262 = call <vilib>:"Simple Error Handler.vi"("error in (no error)"=w485) -> ("error out"=w484:errorcluster)  [unwired: 4 in, 4 out]
                n263 = call <vilib>:"Clear Errors.vi"("error in (no error)"=w484) -> ()  [unwired: 5 in, 2 out]
                n264 = local write "stop 2"(TRUE) -> ()
              }
            }
            n265 = local read "stop 2"() -> (w410:bool)
          }
        }
        event "Aceptar": Mouse Down {
          n266 = event-data() -> ()  [unwired: 1 in, 8 out]
          n267 = while {
            tunnel: "Clave" -> [w503]
            tunnel: "Nombre" -> [w502]
            shift-right: [w500] -> _
            shift-left: Control_2maqinestaaleluya."Control" -> [w501]
            stop <- w499 stop-if-true
            n268 = case shown="\"Aceptar\"" w501 {
              tunnel: w503 -> [_ w512 w519 w531 w568]
              tunnel: w502 -> [_ w511 _ _ w567]
              tunnel: [w506 w509 w517 w530 _] -> w500
              frame "Control", Default {
                n269 = local write "stop 4"(FALSE) -> ()
                n270 = local read "OK Button"() -> (w505:bool)
                n271 = Select(t=Control_2maqinestaaleluya."V.Usuario/Contraseña", s=w505, f=Control_2maqinestaaleluya."Control") -> (s? t:f=w506:T4)
              }
              frame "V.Usuario/Contraseña" {
                n272 = Not Equal?(x=w512, y=w511) -> (x != y?=w510:bool)
                n273 = case shown="True" w510 {
                  tunnel: [Control_2maqinestaaleluya."Control" Control_2maqinestaaleluya."V.Entre 8 y 16"] -> w509
                  frame False {
                    n274 = local write "stop 4"(TRUE) -> ()
                    n275 = One Button Dialog(message="Usuario o Contraseña\n        Incorrectos") -> ()  [unwired: 1 in, 1 out]
                  }
                  frame True {
                  }
                }
              }
              frame "V.Entre 8 y 16" {
                n276 = String To Byte Array(string=w519) -> (unsigned byte array=w520:u8[])
                n277 = Array Size(array=w520) -> (size(s)=w521:i32)
                n278 = Greater Or Equal?(x=w521, y=8) -> (x >= y?=w524:bool)
                n279 = Less Or Equal?(x=w521, y=16) -> (x <= y?=w525:bool)
                n280 = And(x=w524, y=w525) -> (x .and. y?=w518:bool)
                n281 = case shown="True" w518 {
                  tunnel: [Control_2maqinestaaleluya."Control" Control_2maqinestaaleluya."V.min y MAY"] -> w517
                  frame False {
                    n282 = One Button Dialog(message="Usuario o Contraseña\n        Incorrectos") -> ()  [unwired: 1 in, 1 out]
                    "stop 4" <- TRUE
                  }
                  frame True {
                  }
                }
              }
              frame "V.min y MAY" {
                n283 = String To Byte Array(string=w531) -> (unsigned byte array=w536:u8[])
                "C.V 2" <- w536
                n284 = Array Size(array=w536) -> (size(s)=w533:i32)
                n285 = for {
                  N: w533 -> [_]
                  tunnel: [w551] -> w535
                  i -> [w551]
                  n286 = local read "C.V 2"() -> (w554:u8[])
                  n287 = Index Array(array=w554, index=w551) -> (element=w553:u8)
                  n288 = In Range and Coerce(upper limit=90, x=w553, lower limit=65) -> (In Range?=w550:bool)  [unwired: 1 out]
                  n289 = In Range and Coerce(upper limit=122, x=w553, lower limit=97) -> (In Range?=w552:bool)  [unwired: 1 out]
                  n290 = case shown="False" w552 {
                    frame False {
                    }
                    frame True {
                      n291 = local read "min"() -> (w564:i32)
                      n292 = Add(x=w564, y=1) -> (x+y=w563:i32)
                      n293 = local write "min"(w563) -> ()
                    }
                  }
                  n294 = case shown="False" w550 {
                    frame False {
                    }
                    frame True {
                      n295 = local read "mayu"() -> (w561:i32)
                      n296 = Add(x=w561, y=1) -> (x+y=w560:i32)
                      n297 = local write "mayu"(w560) -> ()
                    }
                  }
                }
                n298 = Subtract(x=w533, y=1) -> (x-y=w534:i32)
                n299 = Equal?(x=w534, y=w535) -> (x = y?=w532:bool)
                n300 = case shown="True" w532 {
                  tunnel: [_ w544] -> w530
                  frame False {
                  }
                  frame True {
                    n301 = local read "mayu"() -> (w538:i32)
                    n302 = local read "min"() -> (w541:i32)
                    n303 = Greater Or Equal?(x=w538, y=1 ("x")) -> (x >= y?=w543:bool)
                    n304 = Greater Or Equal?(x=w541, y=1 ("x")) -> (x >= y?=w542:bool)
                    n305 = And(x=w543, y=w542) -> (x .and. y?=w545:bool)
                    n306 = case shown="False" w545 {
                      tunnel: [Control_2maqinestaaleluya."Control" Control_2maqinestaaleluya."Aceptar"] -> w544
                      frame False {
                        n307 = local write "stop 4"(TRUE) -> ()
                        n308 = One Button Dialog(message="Usuario o Contraseña\n        Incorrectos") -> ()  [unwired: 1 in, 1 out]
                      }
                      frame True {
                      }
                    }
                  }
                }
              }
              frame "Aceptar" {
                n309 = Concatenate Strings(w567, "\t", w568) -> (w581:string)
                n310 = Concatenate Strings("\n", w581) -> (w586:string)
                n311 = call <vilib>:"Application Directory.vi"() -> ("Application Directory"=w579:path)
                n312 = Build Path(base path=w579, name or relative path="Nuevo documento de texto.txt") -> (appended path=w580:path)
                n313 = Open/Create/Replace File(file path (use dialog)=w580, operation (0:open)=T1."open", access (0:read/write)=enum16{"read/write", "read-only", "write-only"}."read/write") -> (refnum out=w577:refnum<file>, error out=w578:errorcluster)  [unwired: 3 in, 1 out]
                n314 = Set File Position(offset (in bytes) (0)=i64 0, refnum=w577, from (0:start)=enum16{"start", "end", "current"}."end", error in=w578) -> (refnum out=w585:refnum<file>, error out=w582:errorcluster)
                n315 = Write to Text File(file (use dialog)=w585, text=w586, error in=w582) -> (refnum out=w584:refnum<file>, error out=w583:errorcluster)  [unwired: 1 in, 1 out]
                n316 = Close File(refnum=w584, error in=w583) -> (error out=w576:errorcluster)  [unwired: 1 out]
                n317 = call <vilib>:"Simple Error Handler.vi"("error in (no error)"=w576) -> ("error out"=w575:errorcluster)  [unwired: 4 in, 4 out]
                n318 = call <vilib>:"Clear Errors.vi"("error in (no error)"=w575) -> ()  [unwired: 5 in, 2 out]
                n319 = local write "stop 4"(TRUE) -> ()
              }
            }
            n320 = local read "stop 4"() -> (w499:bool)
          }
        }
        event "Borrar": Mouse Down {
          w598 = "" ("format string")
          n321 = event-data() -> ()  [unwired: 1 in, 8 out]
          n322 = Get File Size(file=w588, error in=w606) -> (refnum out=w592:refnum<file>, 0:w591:errorcluster)  [unwired: 1 out]
          n323 = Set File Position(offset (in bytes) (0)=i64 0, refnum=w592, error in=w591) -> (refnum out=w589:refnum<file>, error out=w590:errorcluster)  [unwired: 1 in]
          n324 = Read from Text File(file (use dialog)=w589, error in=w590) -> (refnum out=w605:refnum<file>, text=w597:string, error out=w604:errorcluster)  [unwired: 2 in, 1 out]
          "text 2" <- w597
          n325 = Spreadsheet String To Array(delimiter (Tab)="\\n", format string=w598, spreadsheet string=w597, array type (2D Dbl)=w598) -> (array=w596:string[][])
          "array 2" <- w596
          n326 = Index Array(array=w596, index (row)=1) -> ()  [unwired: 1 in, 1 out]
          n327 = Index Array(array=w596, index (row)=0) -> (element=w595:string[])  [unwired: 1 in]
          n328 = Index Array(array=w595, index=0) -> (element=w593:string)
          n329 = String To Byte Array(string=w593) -> (unsigned byte array=w611:u8[])
          n330 = Array Size(array=w611) -> (size(s)=w612:i32)
          n331 = for {
            N: w612 -> [_]
            tunnel: [w617] -> w610 if=w617
            tunnel: [w616] -> w609
            tunnel: [w615] -> w608
            tunnel: [w614] -> w607
            i -> [w614]
            stop <- w617 stop-if-true
            n332 = local read "array 2"() -> (w613:string[][])
            n333 = Index Array(array=w613, index (row)=w614, index (col)=0 ("disabled index (col)")) -> (element=w626:string)
            n334 = Match Pattern(string=w626, regular expression="\t") -> (before substring=w622:string, match substring=→"match substring 3":string, after substring=w623:string)  [unwired: 1 in, 1 out]
            "before substring 3" <- w622
            "after substring 3" <- w623
            n335 = local read "Clave/ingress"() -> (w615:string)
            n336 = local read "Usua/Ingress"() -> (w616:string)
            n337 = Equal?(x=w622, y=w616) -> (x = y?=w621:bool)
            n338 = Equal?(x=w623, y=w615) -> (x = y?=w620:bool)
            n339 = And(x=w621, y=w620) -> (x .and. y?=w619:bool)
            n340 = Equal?(x=w619, y=TRUE) -> (x = y?=w617:bool)
          }
          n341 = case shown="True" w610 {
            tunnel: w609 -> [_ w642]
            tunnel: w608 -> [_ w643]
            tunnel: w607 -> [_ w628]
            tunnel: w605 -> [_ w636]
            tunnel: [_ w632] -> w602
            tunnel: [_ w630] -> w603
            tunnel: w604 -> [_ w635]
            tunnel: w604 -> [_ _]
            frame False {
            }
            frame True {
              n342 = for {
                N: w628 -> [_]
                tunnel: w643 -> [w650]
                tunnel: w642 -> [w652]
                tunnel: [w646] -> w641
                i -> [w645]
                n343 = Concatenate Strings(w652, "\t", w650) -> (w648:string)
                n344 = Concatenate Strings("\r\n", w648) -> (w644:string)
                n345 = Insert Into Array(array="Usuarios D/B", index=w645, new element=w644) -> (w646:string[])
              }
              n346 = local read "array 2"() -> (w634:string[][])
              n347 = Delete From Array(array=w634, index (row)=w628) -> (array with subset deleted=w640:string[][])  [unwired: 2 in, 1 out]
              "array w/ subset deleted" <- w640
              n348 = Array To Spreadsheet String(array=w640, 3:"" ("format string")) -> (spreadsheet string=w629:string)  [unwired: 1 in]
              "spreadsheet string" <- w629
              n349 = Write to Text File(file (use dialog)=w636, text=w629, error in=w635) -> (refnum out=w633:refnum<file>, error out=w637:errorcluster)  [unwired: 1 in, 1 out]
              n350 = Set File Size(4:w637, 6:i64 0 ("size (in bytes)"), 7:w633) -> (0:w631:errorcluster, 3:w632:refnum<file>)
              n351 = local write "Usuarios D/B"(w641) -> ()
              n352 = Write to Text File(text=w629, error in=w631) -> (error out=w630:errorcluster)  [unwired: 2 in, 2 out]
            }
          }
        }
      }
    }
    n353 = Close File(refnum=w345, error in=w346) -> ()  [unwired: 2 out]
  }
  n354 = Close File(refnum=w17, error in=w18) -> (error out=w20:errorcluster)  [unwired: 1 out]
  n355 = Close File(refnum=w3, error in=w2) -> (error out=w15:errorcluster)  [unwired: 1 out]
  n356 = call <vilib>:"Simple Error Handler.vi"("error in (no error)"=w20) -> ("error out"=w19:errorcluster)  [unwired: 4 in, 4 out]
  n357 = call <vilib>:"Simple Error Handler.vi"("error in (no error)"=w15) -> ("error out"=w16:errorcluster)  [unwired: 4 in, 4 out]
  n358 = call <vilib>:"Clear Errors.vi"("error in (no error)"=w19) -> ()  [unwired: 5 in, 2 out]
  n359 = call <vilib>:"Clear Errors.vi"("error in (no error)"=w16) -> ()  [unwired: 5 in, 2 out]
  "Tab Control" <- Controlaleluya."Loguin"
  "mayu" <- 0 ("mayu")
  "min" <- 0 ("min")
  "OK Button 2" <- TRUE
  "Tab Control 2" <- Controlaleluya."Loguin"
  "mayu 2" <- 0 ("mayu")
  "min 2" <- 0 ("min")
  "OK Button 3" <- TRUE
  "OK Button" <- TRUE
